vi "labview_target.vi"() -> ()   [LabVIEW 2023]
doc: "You can use the System Exec VI to call command line utilities that return standard output to the command shell. You also can call interactive applications that you intend to launch using System Exec, but interact with using the UI of the executable."
uses:
  <vilib>/Math Plots/3D Math Plots/3D Scatter/3D Scatter XCtrl/3D Scatter.xctl
  <vilib>/Math Plots/3D Math Plots/3D Scatter/3D Scatter Datatype/Public/Plot Helper (Vector).vi
  <vilib>/Math Plots/3D Math Plots/3D Scatter/3D Scatter Datatype/3D Scatter Datatype.lvclass
panel:
  out "LED ID":i32
  out "3D Scatter":refnum<class "3D Plot Datatype.lvclass">[](xcontrol)
  out "Z position (mm)":string
  out "X position (mm)":string
  out "Y position (mm)":string
  out "Frame":string
  out "data out":string
  in  "Server IP address":string="192.168.50.19"
  in  "Stop Button":bool
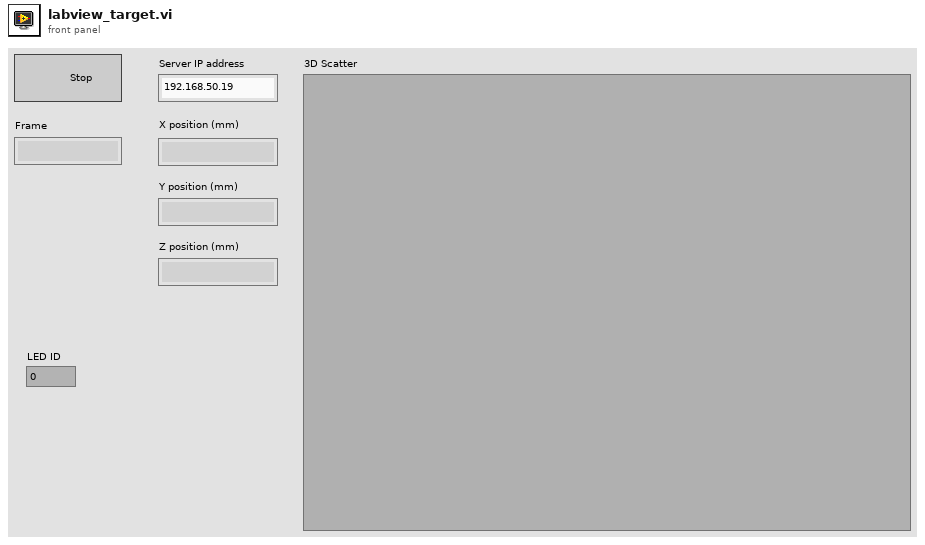
[diagram p1: front panel]
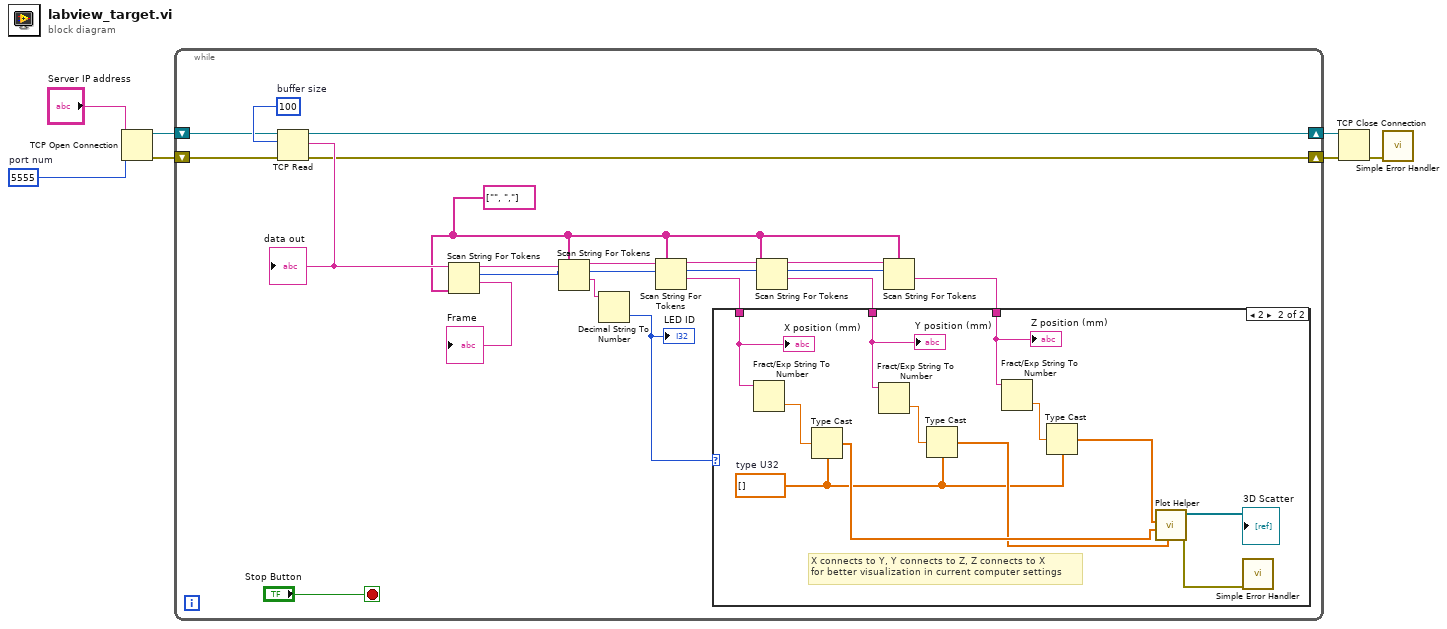
[diagram p0: block diagram]
diagram:
  w7 = 5555  # port num
  n1 = TCP Open Connection(address="Server IP address", remote port or service name=w7) -> (connection ID=w4:refnum<k5>, error out=w1:errorcluster)  [unwired: 3 in]
  n2 = while {
    shift-right: [w23] -> w2
    shift-left: w1 -> [w27]
    shift-right: [w28] -> w6
    shift-left: w4 -> [w26]
    stop <- "Stop Button" stop-if-true
    w17 = string[] ["", ","]
    w29 = 100  # buffer size
    n3 = TCP Read(connection ID=w26, bytes to read=w29, error in (no error)=w27) -> (connection ID out=w28:refnum<k5>, data out=w24:string, error out=w23:errorcluster)  [unwired: 2 in]
    "data out" <- w24
    n4 = Scan String For Tokens(6:w17, 9:w24) -> (1:→"Frame":string, 2:w20:i32, 3:w21:string)  [unwired: 4 in, 1 out]
    n5 = Scan String For Tokens(6:w17, 8:w20, 9:w21) -> (1:w9:string, 2:w18:i32, 3:w19:string)  [unwired: 3 in, 1 out]
    n6 = Decimal String To Number(string=w9) -> (number=w8:i32)  [unwired: 2 in, 1 out]
    "LED ID" <- w8
    n7 = Scan String For Tokens(6:w17, 8:w18, 9:w19) -> (1:w10:string, 2:w16:i32, 3:w15:string)  [unwired: 3 in, 1 out]
    n8 = Scan String For Tokens(6:w17, 8:w16, 9:w15) -> (1:w12:string, 2:w14:i32, 3:w13:string)  [unwired: 3 in, 1 out]
    n9 = Scan String For Tokens(6:w17, 8:w14, 9:w13) -> (1:w11:string)  [unwired: 3 in, 3 out]
    n10 = case shown="2" w8 {
      tunnel: w12 -> [_ w35]
      tunnel: w11 -> [_ w33]
      tunnel: w10 -> [_ w30]
      frame 0, Default {
      }
      frame 2 {
        w31 = dbl[] []  # type U32
        # "X connects to Y, Y connects to Z, Z connects to X\nfor better visualization in current computer settings"
        n11 = Fract/Exp String To Number(string=w30) -> (number=w36:dbl)  [unwired: 3 in, 1 out]
        n12 = Type Cast(type=w31, x=w36) -> (*(type *) &x=w39:dbl[])
        n13 = Fract/Exp String To Number(string=w35) -> (number=w34:dbl)  [unwired: 3 in, 1 out]
        n14 = Type Cast(type=w31, x=w34) -> (*(type *) &x=w38:dbl[])
        n15 = Fract/Exp String To Number(string=w33) -> (number=w32:dbl)  [unwired: 3 in, 1 out]
        n16 = Type Cast(type=w31, x=w32) -> (*(type *) &x=w37:dbl[])
        n17 = call-poly <vilib>:"Plot Helper.vi"("z vector"=w38, "y vector"=w39, "x vector"=w37) -> ("error out"=w41:errorcluster, "3D Plot lvclass Array out"=→"3D Scatter":refnum<class "3D Plot Datatype.lvclass">[])  [unwired: 3 in, 4 out]
        n18 = call <vilib>:"Simple Error Handler.vi"("error in (no error)"=w41) -> ()  [unwired: 2 in, 7 out]
        "Y position (mm)" <- w35
        "X position (mm)" <- w30
        "Z position (mm)" <- w33
      }
    }
  }
  n19 = TCP Close Connection(connection ID=w6, error in (no error)=w2) -> (error out=w5:errorcluster)  [unwired: 1 in, 1 out]
  n20 = call <vilib>:"Simple Error Handler.vi"("error in (no error)"=w5) -> ()  [unwired: 2 in, 7 out]
